vi "Export single clipboard - LDLTS cluster.vi"(5 "Error In":errorcluster, 6 "Workspace":path, 8 "LDLTS measurement":T1={"Name"="", "Comment"="", "Time"=timestamp(0 s since 1904-01-01), "Folder"=path "", "LDLTS properties"={"T"=0.0, "Test signal"=0.0, "Test frequency"=0.0, "Bandwidth"=0.0, "Averaging"=0.0, "Vbias"=0.0, "Vpulse"=0.0, "pulse length"=0.0, "Pulse 2"=FALSE, "Vpulse 2"=0.0, "pulse length 2"=0.0, "I range"=-2.0, "V range"=10.0, "Sampling rate"=0.0, "Acq. delay"=0.0, "Sampling time"=0.0}, "GUID"=""} {"LDLTS properties"."V range" items=["10mV"=0.01, "100mV"=0.1, "1V"=1.0, "10V"=10.0]; "LDLTS properties"."I range" items=["100nA"=-7.0, "1µA"=-6.0, "10µA"=-5.0, "100µA"=-4.0, "1mA"=-3.0, "10mA"=-2.0]}) -> (0 "Error Out":errorcluster)   [LabVIEW 2019]
doc: "Handles export of measurement (identified by a tag) to a .dat file, displays a GUI window"
uses:
  Type defs/LDLTS properties Type Def.ctl
  Type defs/LDLTS measurement Type Def.ctl
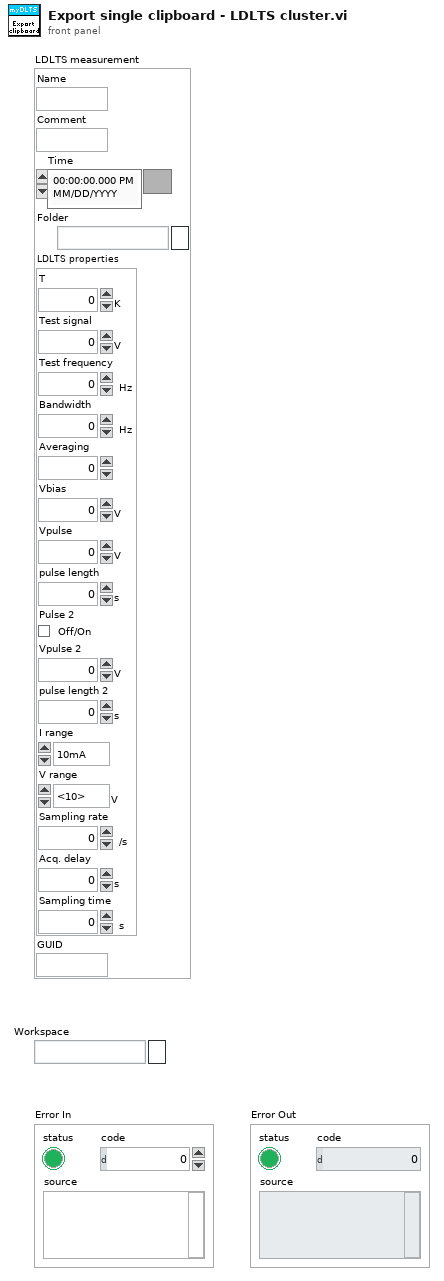
[diagram p1: front panel]
types:
  T1 = typedef "LDLTS measurement Type Def.ctl" = cluster{"Name":string, "Comment":string, "Time":timestamp, "Folder":path, "LDLTS properties":T2, "GUID":string}
  T2 = typedef "LDLTS properties Type Def.ctl" = cluster{"T":dbl[unit], "Test signal":dbl[unit], "Test frequency":dbl[unit], "Bandwidth":dbl[unit], "Averaging":dbl, "Vbias":dbl[unit], "Vpulse":dbl[unit], "pulse length":dbl[unit], "Pulse 2":bool, "Vpulse 2":dbl[unit], "pulse length 2":dbl[unit], "I range":dbl, "V range":dbl[unit], "Sampling rate":dbl[unit], "Acq. delay":dbl[unit], "Sampling time":dbl[unit]}
  T3 = cluster{"Name":string, "Files":path[], "Header":string[][]}
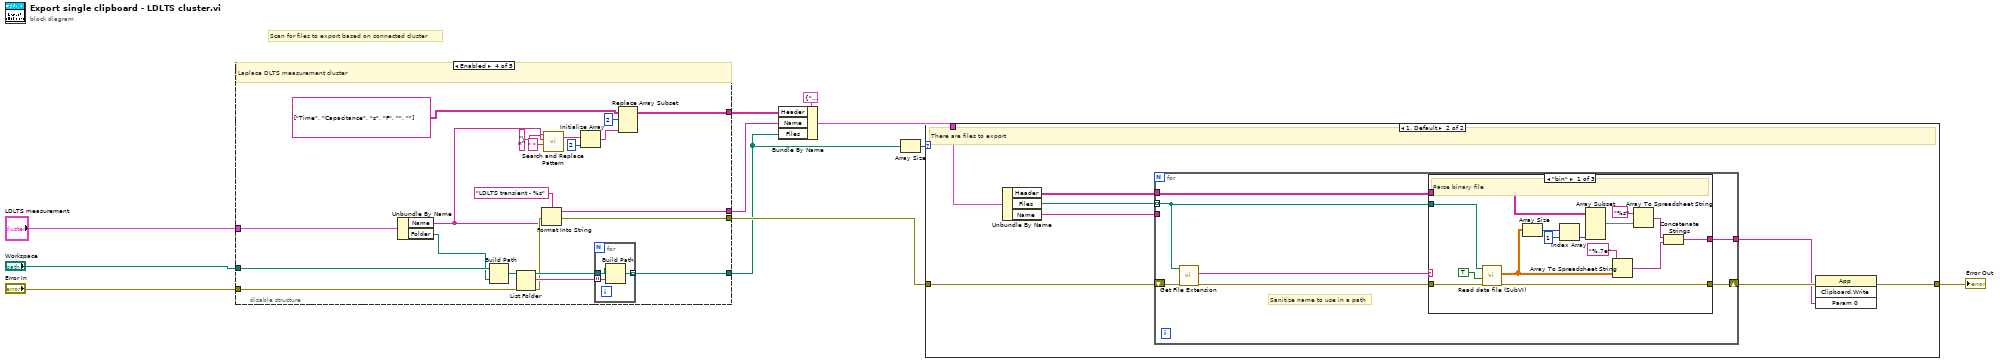
[diagram p0: block diagram]
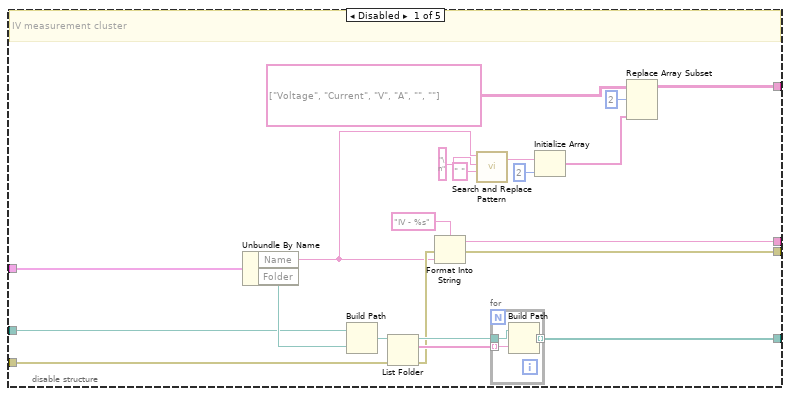
[diagram p2: hidden frame]
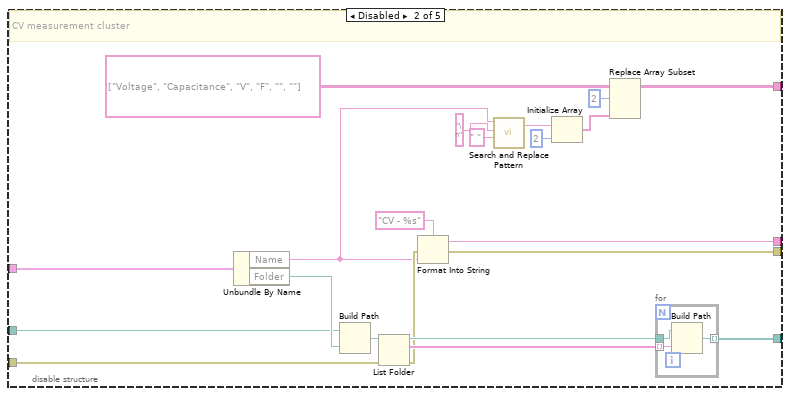
[diagram p3: hidden frame]
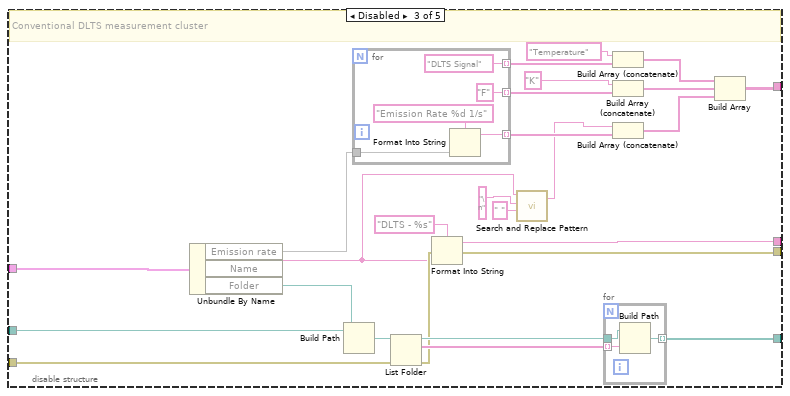
[diagram p4: hidden frame]
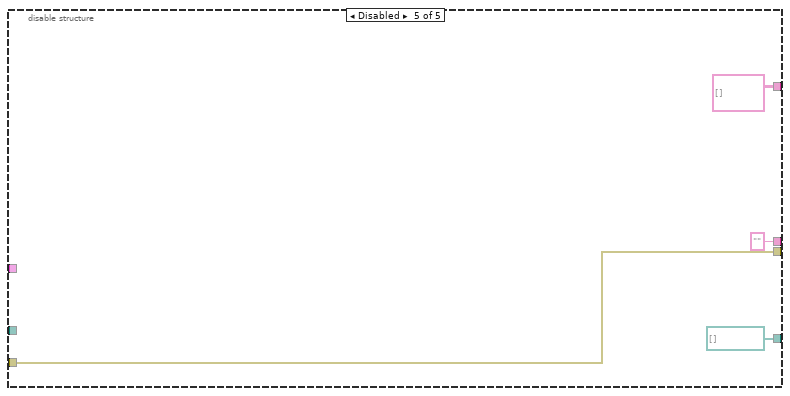
[diagram p5: hidden frame]
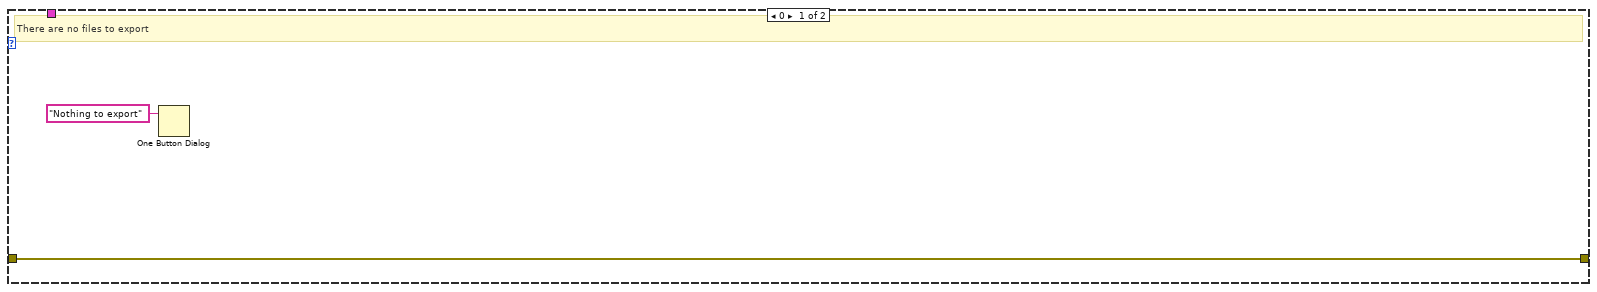
[diagram p6: hidden frame]
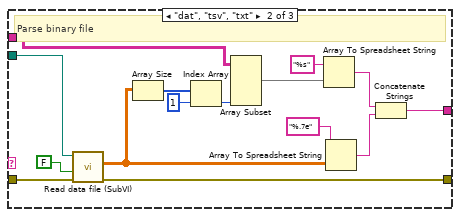
[diagram p7: hidden frame]
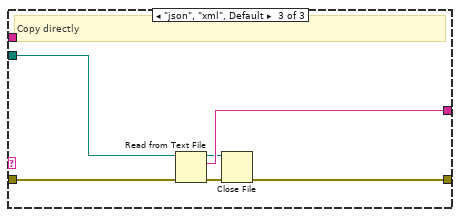
[diagram p8: hidden frame]
diagram:
  # "Scan for files to export based on connected cluster"
  n1 = disable-structure shown="Enabled" {
    disable-tunnel: [w19 w39 w70 w97 string[][] []] -> w6
    disable-tunnel: [w26 w50 w69 w109 ""] -> w5
    disable-tunnel: [w25 w49 w68 w108 w119] -> w3
    disable-tunnel: [w24 w48 w67 w107 path[] []] -> w2
    disable-tunnel: "Workspace" -> [w23 w46 w65 w105 _]
    disable-tunnel: "Error In" -> [w22 w47 w66 w106 w119]
    disable-tunnel: "LDLTS measurement" -> [w21 w45 w64 w103 _]
    frame Disabled {
      # "IV measurement cluster"
      n2 = Unbundle By Name(w21) -> ("Name"=w12:string, "Folder"=w31:path)
      n3 = Build Path(base path=w23, name or relative path=w31) -> (appended path=w29:path)
      n4 = List Folder(path=w29, error in=w22) -> (path out=w28:path, filenames=w30:string[], error out=w27:errorcluster)  [unwired: 2 in, 1 out]
      n5 = Format Into String(format string="IV - %s", error in=w27, w12) -> (resulting string=w26:string, error out=w25:errorcluster)  [unwired: 1 in]
      n6 = call <vilib>:"Search and Replace Pattern.vi"("string"=w12, "regular expression (\"\")"="\n" ("regular expression (\"\")"), "replace string (\"\")"=" " ("replace string (\"\")")) -> ("result string"=w17:string)  [unwired: 2 in, 1 out]
      n7 = for {
        tunnel: w28 -> [w35]
        tunnel: [w34] -> w24 mode=indexing
        tunnel: w30 -> [w33] mode=indexing
        n8 = Build Path(base path=w35, name or relative path=w33) -> (appended path=w34:path)
      }
      n9 = Initialize Array(w17, 2 ("dimension size")) -> (w13:string[])
      n10 = Replace Array Subset(array=string[][] [["Voltage", "Current"], ["V", "A"], ["", ""]], new element=w13, index (row)=2) -> (w19:string[][])  [unwired: 1 in]
    }
    frame Disabled {
      # "CV measurement cluster"
      n11 = Unbundle By Name(w45) -> ("Name"=w37:string, "Folder"=w55:path)
      n12 = Build Path(base path=w46, name or relative path=w55) -> (appended path=w53:path)
      n13 = List Folder(path=w53, error in=w47) -> (path out=w52:path, filenames=w54:string[], error out=w51:errorcluster)  [unwired: 2 in, 1 out]
      n14 = Format Into String(format string="CV - %s", error in=w51, w37) -> (resulting string=w50:string, error out=w49:errorcluster)  [unwired: 1 in]
      n15 = call <vilib>:"Search and Replace Pattern.vi"("string"=w37, "regular expression (\"\")"="\n" ("regular expression (\"\")"), "replace string (\"\")"=" " ("replace string (\"\")")) -> ("result string"=w43:string)  [unwired: 2 in, 1 out]
      n16 = Initialize Array(w43, 2 ("dimension size")) -> (w44:string[])
      n17 = Replace Array Subset(array=string[][] [["Voltage", "Capacitance"], ["V", "F"], ["", ""]], new element=w44, index (row)=2) -> (w39:string[][])  [unwired: 1 in]
      n18 = for {
        tunnel: w52 -> [w59]
        tunnel: [w58] -> w48 mode=indexing
        tunnel: w54 -> [w57] mode=indexing
        n19 = Build Path(base path=w59, name or relative path=w57) -> (appended path=w58:path)
      }
    }
    frame Disabled {
      # "Conventional DLTS measurement cluster"
      n20 = Unbundle By Name(w64) -> ("Emission rate"=w71, "Name"=w62:string, "Folder"=w72:path)
      n21 = Build Path(base path=w65, name or relative path=w72) -> (appended path=w82:path)
      n22 = for {
        tunnel: w71 -> [w90]
        tunnel: [w88] -> w78 mode=indexing
        tunnel: ["DLTS Signal"] -> w76 mode=indexing
        tunnel: ["F"] -> w77 mode=indexing
        n23 = Format Into String(format string="Emission Rate %d 1/s", w90) -> (resulting string=w88:string)  [unwired: 2 in, 1 out]
      }
      n24 = List Folder(path=w82, error in=w66) -> (path out=w83:path, filenames=w84:string[], error out=w81:errorcluster)  [unwired: 2 in, 1 out]
      n25 = Format Into String(format string="DLTS - %s", error in=w81, w62) -> (resulting string=w69:string, error out=w68:errorcluster)  [unwired: 1 in]
      n26 = call <vilib>:"Search and Replace Pattern.vi"("string"=w62, "regular expression (\"\")"="\n" ("regular expression (\"\")"), "replace string (\"\")"=" " ("replace string (\"\")")) -> ("result string"=w60:string)  [unwired: 2 in, 1 out]
      n27 = for {
        tunnel: w83 -> [w93]
        tunnel: [w92] -> w67 mode=indexing
        tunnel: w84 -> [w91] mode=indexing
        n28 = Build Path(base path=w93, name or relative path=w91) -> (appended path=w92:path)
      }
      n29 = Build Array (concatenate)("Temperature", w76) -> (w73:string[])
      n30 = Build Array (concatenate)("K", w77) -> (w74:string[])
      n31 = Build Array (concatenate)(w60, w78) -> (w75:string[])
      n32 = Build Array(w73, w74, w75) -> (w70:string[][])
    }
    frame Enabled {
      # "Laplace DLTS measurement cluster"
      n33 = Unbundle By Name(w103) -> ("Name"=w96:string, "Folder"=w104:path)
      n34 = Build Path(base path=w105, name or relative path=w104) -> (appended path=w112:path)
      n35 = List Folder(path=w112, error in=w106) -> (path out=w111:path, filenames=w113:string[], error out=w110:errorcluster)  [unwired: 2 in, 1 out]
      n36 = Format Into String(format string="LDLTS transient - %s", error in=w110, w96) -> (resulting string=w109:string, error out=w108:errorcluster)  [unwired: 1 in]
      n37 = call <vilib>:"Search and Replace Pattern.vi"("string"=w96, "regular expression (\"\")"="\n" ("regular expression (\"\")"), "replace string (\"\")"=" " ("replace string (\"\")")) -> ("result string"=w102:string)  [unwired: 2 in, 1 out]
      n38 = Initialize Array(w102, 2 ("dimension size")) -> (w100:string[])
      n39 = for {
        tunnel: w111 -> [w117]
        tunnel: [w116] -> w107 mode=indexing
        tunnel: w113 -> [w115] mode=indexing
        n40 = Build Path(base path=w117, name or relative path=w115) -> (appended path=w116:path)
      }
      n41 = Replace Array Subset(array=string[][] [["Time", "Capacitance"], ["s", "F"], ["", ""]], new element=w100, index (row)=2) -> (w97:string[][])  [unwired: 1 in]
    }
    frame Disabled {
    }
  }
  n42 = Bundle By Name(cluster=T3 {"Name"="", "Files"=[], "Header"=[]} ("output cluster"), "Header"=w6, "Name"=w5, "Files"=w2) -> (w4:T3)
  n43 = Array Size(array=w2) -> (size(s)=w11:i32)
  n44 = case shown="1, Default" w11 {
    tunnel: w3 -> [w122 w127]
    tunnel: [w122 w125] -> w9
    tunnel: w4 -> [_ w131]
    frame 0 {
      # "There are no files to export"
      n45 = One Button Dialog(message="Nothing to export") -> ()  [unwired: 1 in, 1 out]
    }
    frame 1, Default {
      # "There are files to export"
      n46 = Unbundle By Name(w131) -> ("Header"=w128:string[][], "Files"=w130:path[], "Name"=w129:string)
      n47 = for {
        tunnel: w130 -> [w135] mode=indexing
        tunnel: w129 -> [_]
        tunnel: w128 -> [w134]
        shift-right: [w136] -> w126
        shift-left: w127 -> [w138]
        tunnel: [w132] -> w124
        # "Sanitize name to use in a path"
        n48 = call <vilib>:"Get File Extension.vi"("error in (no error)"=w138, "file"=w135) -> ("error out"=w133:errorcluster, "lowercase file extension"=w137:string)  [unwired: 5 in, 3 out]
        n49 = case shown="\"bin\"" w137 {
          tunnel: w133 -> [w151 w166 w174]
          tunnel: [w148 w163 w170] -> w136
          tunnel: w135 -> [w153 w168 w169]
          tunnel: w134 -> [w141 w156 _]
          tunnel: [w145 w160 w173] -> w132
          frame "bin" {
            # "Parse binary file"
            n50 = call "Read data file (SubVI).vi"("error in"=w151, "Binary"=TRUE, "file path in"=w153) -> ("error out"=w148:errorcluster, "2D data"=w139:dbl[][])  [unwired: 6 in, 1 out]
            n51 = Array Size(array=w139) -> (size(s)=w144:i32[])
            n52 = Index Array(array=w144, index=1) -> (element=w143:i32)
            n53 = Array Subset(array=w141, length (col)=w143) -> (w140:string[][])  [unwired: 3 in]
            n54 = Array To Spreadsheet String(array=w139, 3:"%.7e" ("format (%.3f)")) -> (spreadsheet string=w146:string)  [unwired: 1 in]
            n55 = Array To Spreadsheet String(array=w140, 3:"%s" ("format string")) -> (spreadsheet string=w147:string)  [unwired: 1 in]
            n56 = Concatenate Strings(w147, w146) -> (w145:string)
          }
          frame "dat", "tsv", "txt" {
            # "Parse binary file"
            n57 = call "Read data file (SubVI).vi"("error in"=w166, "Binary"=FALSE, "file path in"=w168) -> ("error out"=w163:errorcluster, "2D data"=w154:dbl[][])  [unwired: 6 in, 1 out]
            n58 = Array Size(array=w154) -> (size(s)=w159:i32[])
            n59 = Index Array(array=w159, index=1) -> (element=w158:i32)
            n60 = Array Subset(array=w156, length (col)=w158) -> (w155:string[][])  [unwired: 3 in]
            n61 = Array To Spreadsheet String(array=w155, 3:"%s" ("format string")) -> (spreadsheet string=w162:string)  [unwired: 1 in]
            n62 = Array To Spreadsheet String(array=w154, 3:"%.7e" ("format (%.3f)")) -> (spreadsheet string=w161:string)  [unwired: 1 in]
            n63 = Concatenate Strings(w162, w161) -> (w160:string)
          }
          frame "json", "xml", Default {
            # "Copy directly"
            n64 = Read from Text File(file (use dialog)=w169, error in=w174) -> (refnum out=w172:refnum<file>, text=w173:string, error out=w171:errorcluster)  [unwired: 2 in, 1 out]
            n65 = Close File(refnum=w172, error in=w171) -> (error out=w170:errorcluster)  [unwired: 1 out]
          }
        }
      }
      n66 = invoke class="App" method="Clipboard.Write"(error in=w126, "Param 0"=w124) -> (error out=w125:errorcluster)  [unwired: 2 in, 3 out]
    }
  }
  "Error Out" <- w9
